vi "Run RT Target VI.vi"(6 "clone#":i32, 8 "doneRef":refnum<vi>, 11 "targetVIref":T1) -> ()   [LabVIEW 2020, in "NI_TargetHelper.lvlib"]
uses:
  <vilib>/TargetSupport/NI_TargetHelper/NI_TargetHelper.lvlib
  <vilib>/TargetSupport/NI_TargetHelper/Instance VIref.ctl
  761217ef-e074-c54f-a090-1f88087bb986.vi
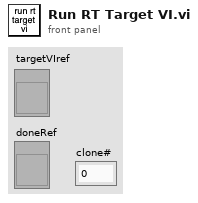
[diagram p1: front panel]
types:
  T1 = typedef "NI_TargetHelper.lvlib/Instance VIref.ctl" = refnum<vi>
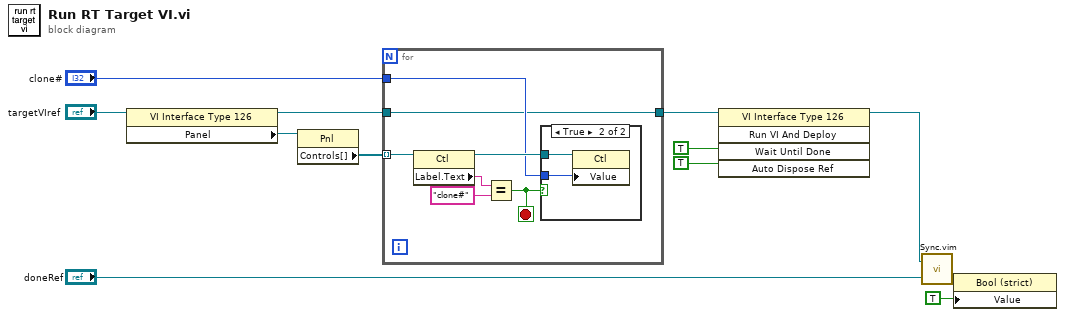
[diagram p0: block diagram]
diagram:
  n1 = property class="VI Interface Type 126"(reference="targetVIref") -> (reference out=w1:T1, "Panel"=w6:refnum<vi>)  [unwired: 1 in, 1 out]
  n2 = property class="Pnl"(reference=w6) -> ("Controls[]"=w5:refnum<vi>[])  [unwired: 1 in, 2 out]
  n3 = for {
    tunnel: w5 -> [w19] mode=indexing
    tunnel: "clone#" -> [w14]
    tunnel: [w13] -> w2
    tunnel: w1 -> [w13]
    stop <- w16 stop-if-true
    n4 = property class="Ctl"(reference=w19) -> (reference out=w15:refnum<vi>, "Label.Text"=w18:string)  [unwired: 1 in, 1 out]
    n5 = Equal?(x=w18, y="clone#") -> (x = y?=w16:bool)
    n6 = case shown="True" w16 {
      tunnel: w15 -> [_ w21]
      tunnel: w14 -> [_ w20]
      frame False {
      }
      frame True {
        n7 = property class="Ctl"(reference=w21, "Value"=w20) -> ()  [unwired: 1 in, 2 out]
      }
    }
  }
  n8 = invoke class="VI Interface Type 126" method="Run VI And Deploy"(reference=w2, "Wait Until Done"=TRUE, "Auto Dispose Ref"=TRUE ("Auto Dispose Reference")) -> (reference out=w7:T1)  [unwired: 2 in, 4 out]
  n9 = call "Sync.vim"("a"=w7, "b"="doneRef") -> ("b'"=w10:refnum<vi>)  [unwired: 24 in, 1 out]
  n10 = property class="Bool (strict)"(reference=w10, "Value"=TRUE) -> ()  [unwired: 1 in, 2 out]
